vi "Query Device ID.vi"(0 "34401 in":refnum<class "34401.lvclass">, 11 "error in (no error)":errorcluster) -> (4 "34401 out":refnum<class "34401.lvclass">, 6 "Model":string, 8 "Serial Number":string, 10 "Firmware":string, 15 "error out":errorcluster)   [LabVIEW 2018, in "34401.lvlib" / "34401.lvclass"]
uses:
  34401.lvclass
  34401.lvclass/34401.ctl
  <instrlib>/Agilent 34401/Agilent 34401.lvlib
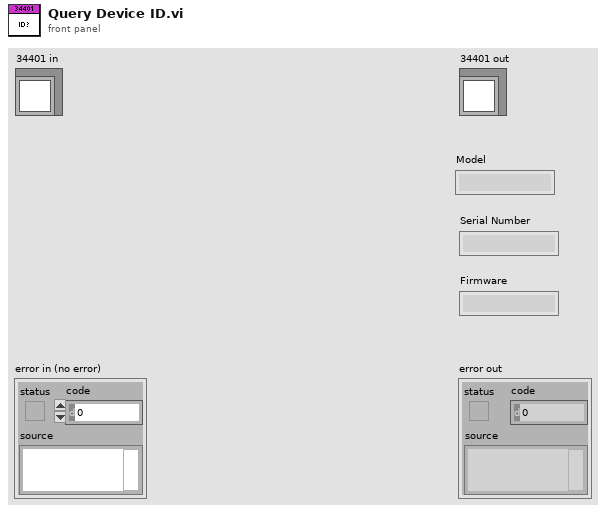
[diagram p1: front panel]
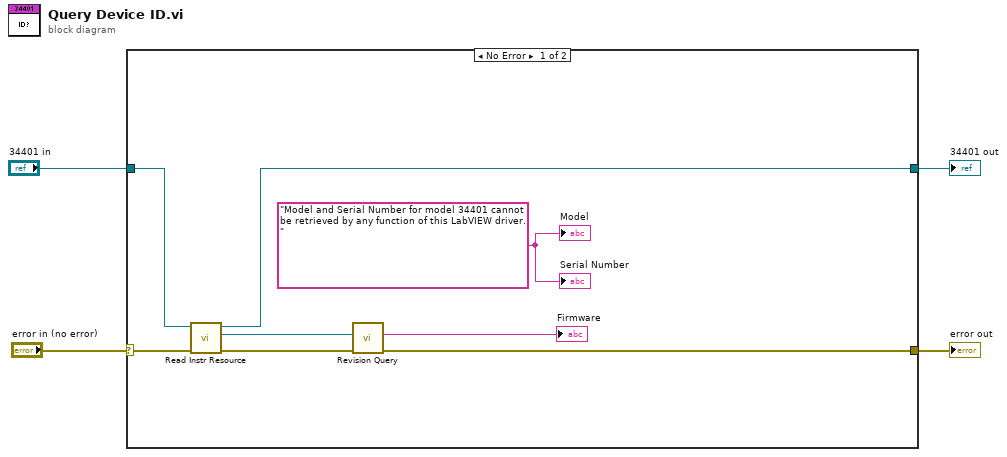
[diagram p0: block diagram]
diagram:
  n1 = case shown="No Error" "error in (no error)" {
    selector: "error in (no error)" -> [w12 w14]
    tunnel: [w6 w14] -> w3
    tunnel: [w8 w13] -> w2
    tunnel: "34401 in" -> [w11 w13]
    frame No Error {
      w5 = "Model and Serial Number for model 34401 cannot be retrieved by any function of this LabVIEW driver."
      n2 = call "Read Instr Resource.vi"("error in (no error)"=w12, "34401 in"=w11) -> ("error out"=w9:errorcluster, "Instr Resource"=w10:refnum<visa-resource-name>, "34401 out"=w8:refnum<class "34401.lvclass">)  [unwired: 7 in]
      n3 = call <instrlib>:"Revision Query.vi"("error in (no error)"=w9, "VISA resource name"=w10) -> ("error out"=w6:errorcluster, "Instrument Firmware Revision"=→"Firmware":string)  [unwired: 6 in, 2 out]
      "Model" <- w5
      "Serial Number" <- w5
    }
    frame Error {
    }
  }
  "error out" <- w3
  "34401 out" <- w2
